vi "niRFUtil MT UTIL AWGN Validate.vi"(5 "Bits Per Symbol (1)":i32=1, 7 "Samples Per Symbol (16)":i32=16, 11 "Waveform In":T1={"x0"=0.0, "dx"=1.0, "y"=[]} caption="input complex waveform" {"y" format="%.2f"; "dx" format="%^.2e"; "x0" format="%^.2e"}) -> (0 "error out":errorcluster)   [LabVIEW 2015, in "niRFUtil.lvlib"]
doc: "This VI validates the inputs for the MT AWGN VI."
uses:
  niRFUtil.lvlib
  Includes/niRFUtil INC Complex Waveform.ctl
  Includes/niRFUtil INC Complex Array.ctl
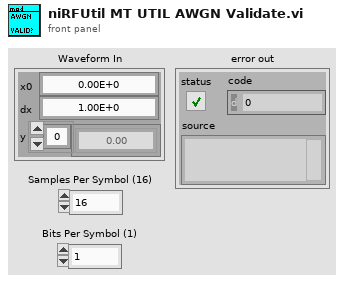
[diagram p1: front panel]
types:
  T1 = typedef "niRFUtil.lvlib/niRFUtil INC Complex Waveform.ctl" = cluster{"x0":dbl, "dx":dbl, "y":T2}
  T2 = typedef "niRFUtil.lvlib/niRFUtil INC Complex Array.ctl" = csg[]
  T3 = cluster{"status":bool, "code":i32, "name":string}[]
  T4 = cluster{"status":bool, "code":i32, "name":string}
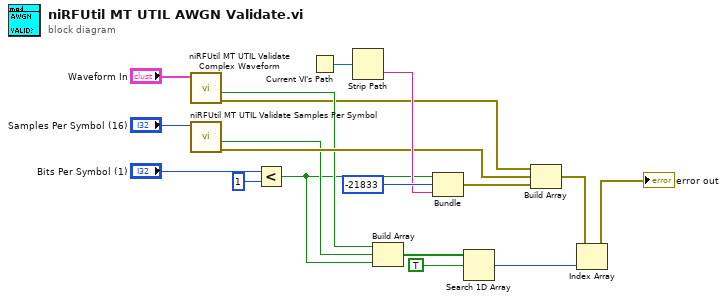
[diagram p0: block diagram]
diagram:
  n1 = call "niRFUtil MT UTIL Validate Complex Waveform.vi"("Waveform In"="Waveform In") -> ("error out"=w6:errorcluster, "error?"=w7:bool)  [unwired: 1 in, 8 out]
  n2 = call "niRFUtil MT UTIL Validate Samples Per Symbol.vi"("Samples Per Symbol"="Samples Per Symbol (16)") -> ("error out"=w9:errorcluster, "error?"=w8:bool)  [unwired: 9 out]
  n3 = Less?(x="Bits Per Symbol (1)", y=1) -> (x < y?=w1:bool)
  n4 = Current VI's Path() -> (path=w18:path)
  n5 = Strip Path(path=w18) -> (name=w10:string)  [unwired: 1 out]
  n6 = Build Array(w7, w8, w1) -> (w17:bool[])
  n7 = Bundle(w1, "code"=-21833, "name"=w10) -> (w11:cluster{bool, "code":i32, "name":string})  [unwired: 1 out]
  n8 = Search 1D Array(1D array=w17, element=TRUE) -> (index of element=w14:i32)  [unwired: 1 out]
  n9 = Build Array(w6, w9, w11) -> (w15:T3)
  n10 = Index Array(array=w15, index=w14) -> (element=→"error out":T4)
